vi "Save Samples.vi"(6 "Type of Feature":string, 8 "error in (no error)":errorcluster, 10 "Images":T1[](array[typedef]), 11 "Destination Folder":path) -> (0 "error out":errorcluster)   [LabVIEW 2013]
uses:
  <vilib>/vision/Image Controls.llb/IMAQ Image.ctl
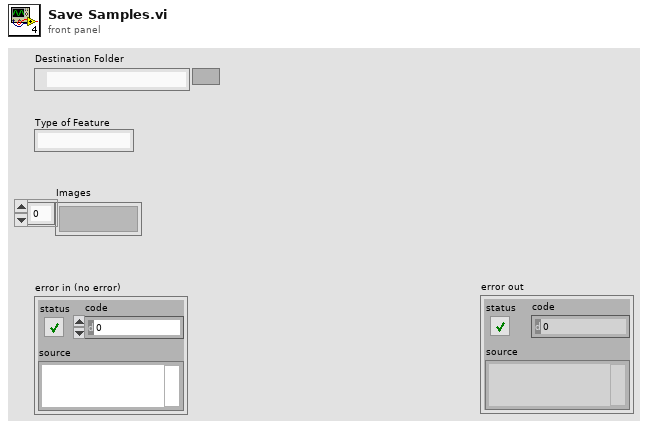
[diagram p1: front panel]
types:
  T1 = typedef "IMAQ Image.ctl" = refnum<image>
  T2 = enum16{"open", "replace", "create", "open or create", "replace or create", "replace or create with confirmation"}
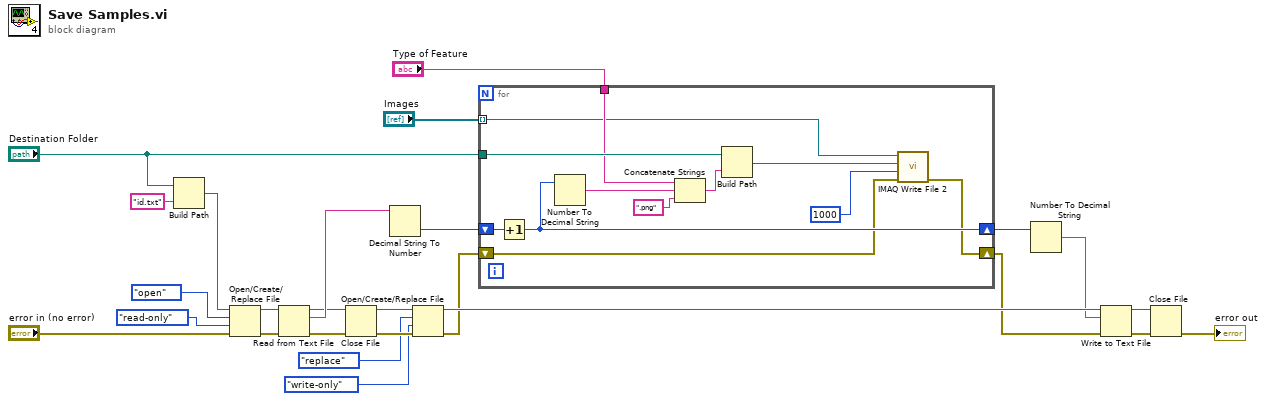
[diagram p0: block diagram]
diagram:
  n1 = Build Path(base path="Destination Folder", name or relative path="id.txt") -> (appended path=w26:path)
  n2 = Open/Create/Replace File(file path (use dialog)=w26, error in="error in (no error)", operation (0:open)=T2."open", access (0:read/write)=enum16{"read/write", "read-only", "write-only"}."read-only") -> (refnum out=w25:refnum<file>, error out=w24:errorcluster)  [unwired: 2 in, 1 out]
  n3 = Read from Text File(file (use dialog)=w25, error in=w24) -> (refnum out=w16:refnum<file>, text=w23:string, error out=w17:errorcluster)  [unwired: 2 in, 1 out]
  n4 = Close File(refnum=w16, error in=w17) -> (path=w14:path, error out=w15:errorcluster)
  n5 = Decimal String To Number(string=w23) -> (number=w22:i32)  [unwired: 2 in, 1 out]
  n6 = Open/Create/Replace File(file path (use dialog)=w14, error in=w15, operation (0:open)=T2."replace", access (0:read/write)=enum16{"read/write", "read-only", "write-only"}."write-only") -> (refnum out=w11:refnum<file>, error out=w4:errorcluster)  [unwired: 2 in, 1 out]
  n7 = for {
    tunnel: "Destination Folder" -> [w34]
    tunnel: "Type of Feature" -> [w33]
    shift-right: [w30] -> w3
    shift-left: w22 -> [w38]
    tunnel: "Images" -> [w29] mode=indexing
    shift-right: [w27] -> w2
    shift-left: w4 -> [w28]
    n8 = Increment(x=w38) -> (x+1=w30:i32)
    n9 = Number To Decimal String(number=w30) -> (decimal integer string=w37:string)  [unwired: 1 in]
    n10 = Concatenate Strings(w33, w37, ".png" ("string")) -> (w35:string)
    n11 = Build Path(base path=w34, name or relative path=w35) -> (appended path=w32:path)
    n12 = call-poly "IMAQ Write File 2"("error in (no error)"=w28, "Image Quality"=u32 1000, "File Path"=w32, "Image"=w29) -> ("error out"=w27:errorcluster)  [unwired: 6 in, 1 out]
  }
  n13 = Number To Decimal String(number=w3) -> (decimal integer string=w1:string)  [unwired: 1 in]
  n14 = Write to Text File(file (use dialog)=w11, text=w1, error in=w2) -> (refnum out=w19:refnum<file>, error out=w18:errorcluster)  [unwired: 1 in, 1 out]
  n15 = Close File(refnum=w19, error in=w18) -> (error out=→"error out":errorcluster)  [unwired: 1 out]
